vi "Get Next.vi"(0 "Conditional in":refnum<class "Case Structure.lvclass">, 1 "Linked List Ref":refnum<data-value>, 5 "Active Unique ID":string, 9 "Active Element Index":i32, 11 "error in (no error)":errorcluster) -> (3 "Linked List Ref out":refnum<data-value>, 4 "Executioner out":refnum<class "Executioner.lvclass">, 6 "Active Unique ID out":string, 8 "Test Executive Ref out":refnum<data-value>, 10 "Active Element Index out":i32, 12 "Found":bool, 13 "Complete":bool, 14 "Stop":bool, 15 "error out":errorcluster)   [LabVIEW 2017, in "Custom Type Test Executive.lvlib" / "Case Structure.lvclass"]
uses:
  <vilib>/gpm_packages/@cs/test-executive/Source/Custom Type Test Executive/Case Structure/Case Structure.lvclass
  C:/Program Files/National Instruments/LabVIEW 2017/vi.lib/gpm_packages/@cs/test-executive/Source/Test Executive/Executioner/Executioner.lvclass
  <vilib>/gpm_packages/@cs/test-executive/Source/Test Executive/Executioner/Executioner.lvclass
  <vilib>/gpm_packages/@cs/linked-list/Source/Linked List/ILinkedList/ILinked List.lvclass
  <vilib>/gpm_packages/@cs/test-executive/Source/Test Executive/ITestExecutive/ITest Executive.lvclass
  <vilib>/gpm_packages/@cs/data-type-serializer/source/Boolean/Boolean.lvclass/Boolean.ctl
  <vilib>/gpm_packages/@cs/run-time-assertions/Source/Assert/Assert.lvclass
  <vilib>/gpm_packages/@cs/data-type-serializer/source/String 1D/String 1D.lvclass/String 1D.ctl
  <vilib>/gpm_packages/@cs/data-type-serializer/source/Assertion 1D/Assertion 1D.lvclass/Assertion 1D.ctl
  <vilib>/gpm_packages/@cs/data-type-serializer/source/I32/I32.lvclass/I32.ctl
  <vilib>/gpm_packages/@cs/data-type-serializer/source/String/String.lvclass/String.ctl
  e3f8ce14-f829-49f2-b732-6c6bdfab1e2b.vi
  37905dbb-9ffa-4c29-9283-9b2d51775808.vi
  3e0f320b-1dba-4963-93ff-3147506816ec.vi
  cd02d659-4998-4fe8-9163-758659dc25cf.vi
  573c41b1-dd6f-44f0-b272-1a8672389ddc.vi
  138538c4-910c-479f-b7e4-eec8342ec67d.vi
  dfe7eb8f-9477-4e6f-83e2-2ac45f956d87.vi
  83fabfc2-d942-454a-aebd-5c424e9e8ceb.vi
  7aa6beab-24c8-424d-8c21-694c569c77be.vi
  c330ebbc-4213-473c-a39d-77c385c7404d.vi
  e43c0b16-206a-4550-822b-640e3cfc4d82.vi
  abd896ed-6152-4a89-b063-422a77b952e5.vi
  <vilib>/gpm_packages/@cs/data-type-serializer/source/Boolean/Boolean.lvclass
  C:/Program Files/National Instruments/LabVIEW 2017/vi.lib/gpm_packages/@cs/data-type-serializer/source/Data Type/Data Type.lvclass
  <vilib>/gpm_packages/@cs/data-type-serializer/source/Assertion 1D/Assertion 1D.lvclass
  <vilib>/gpm_packages/@cs/data-type-serializer/source/String 1D/String 1D.lvclass
  <vilib>/gpm_packages/@cs/data-type-serializer/source/I32/I32.lvclass
  <vilib>/gpm_packages/@cs/data-type-serializer/source/String/String.lvclass
  <vilib>/gpm_packages/@cs/linked-list/Source/Linked List/Linked List Ref/Linked List Ref.lvclass
  <vilib>/gpm_packages/@cs/test-executive/Source/Test Executive/Case Structure/Case Structure.lvclass
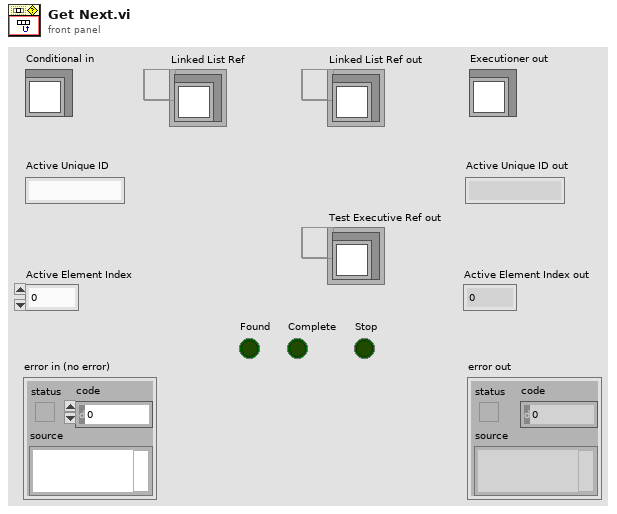
[diagram p1: front panel]
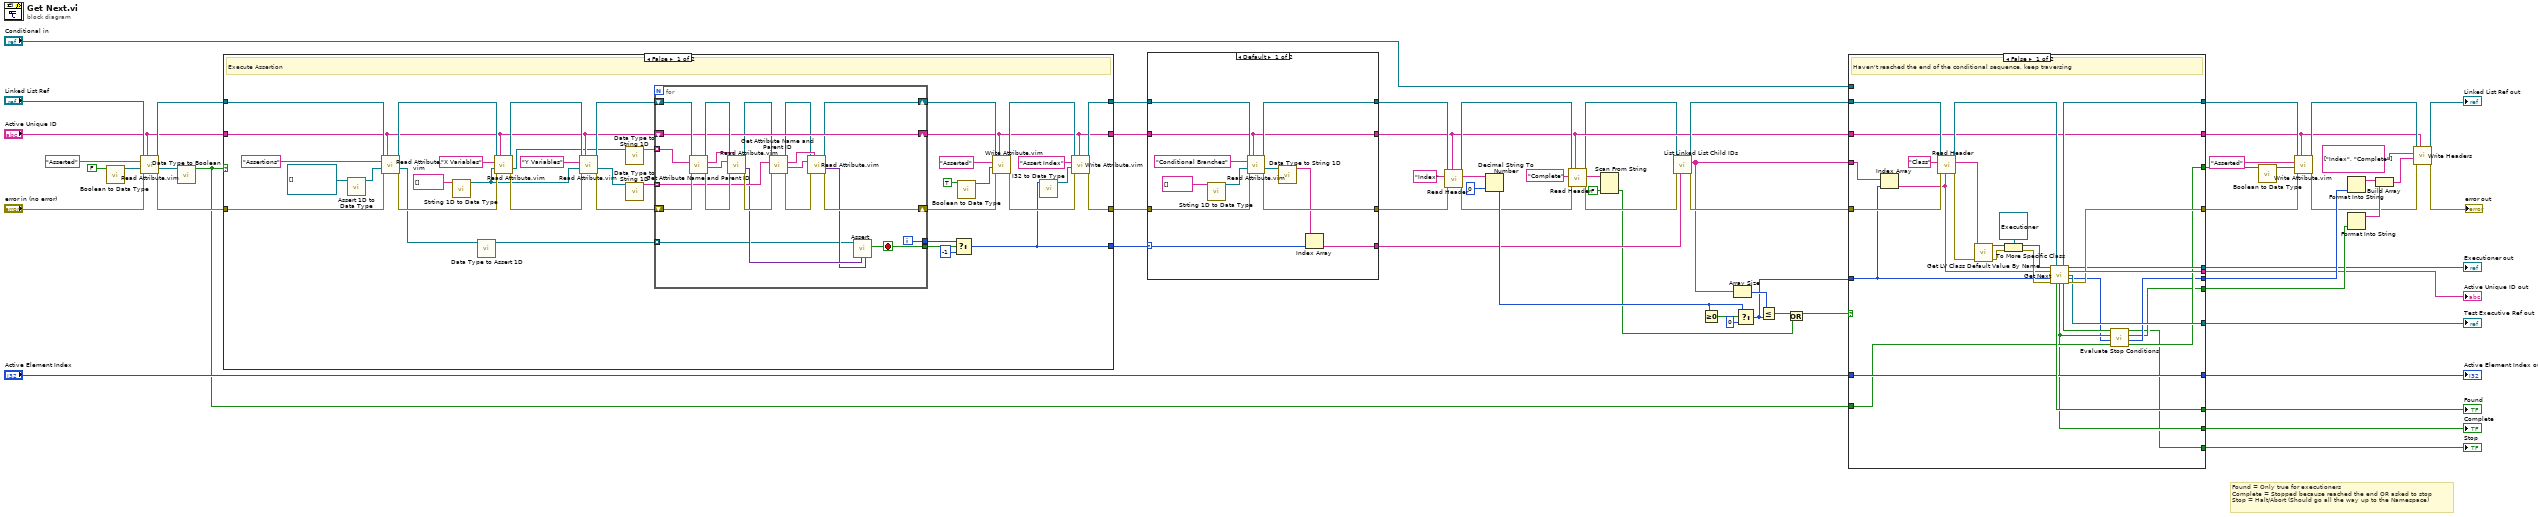
[diagram p0: block diagram]
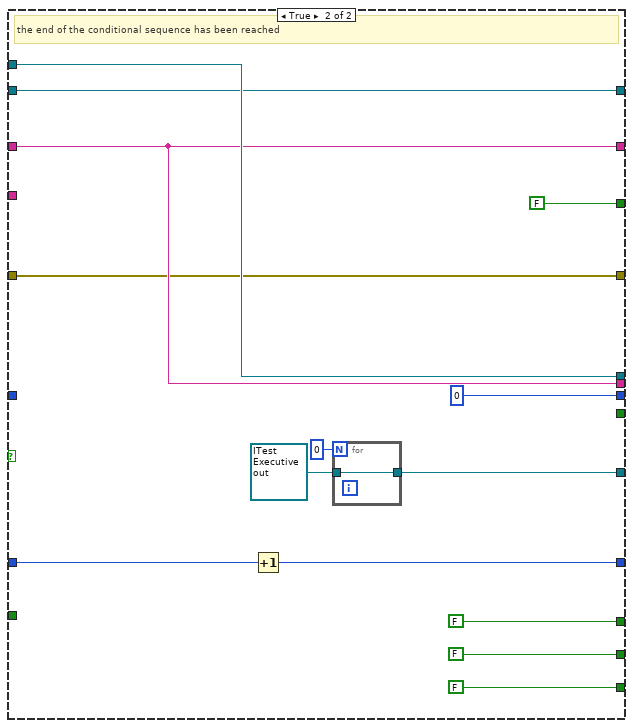
[diagram p2: hidden frame]
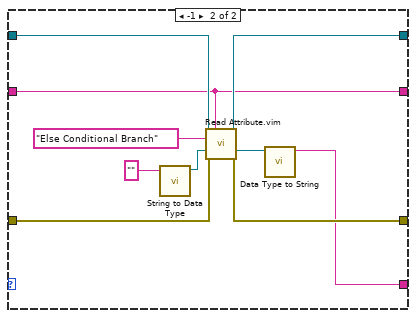
[diagram p3: hidden frame]
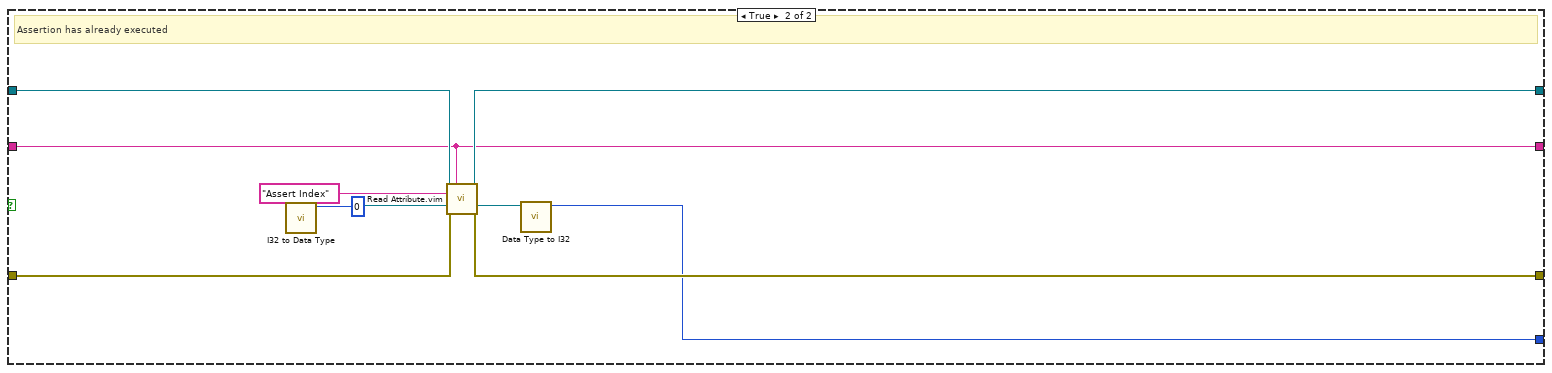
[diagram p4: hidden frame]
diagram:
  # "Found = Only true for executioners\nComplete = Stopped because reached the end OR asked to stop\nStop = Halt/Abort (Should go all the way up to the Namespace)"
  n1 = call <vilib>:"Boolean to Data Type.vi"("Boolean"=FALSE) -> ("Boolean out"=w5:refnum<class "Boolean.lvclass">)  [unwired: 9 in, 1 out]
  n2 = call "Read Attribute.vim"("Linked List Ref"="Linked List Ref", "Linked List ID"="Active Unique ID", "Attribute Name"="Asserted", "Type"=w5, "error in (no error)"="error in (no error)") -> ("Linked List Ref out"=w63:refnum<data-value>, "Attribute"=w4:refnum<class "Boolean.lvclass">, "error out"=w62:errorcluster)  [unwired: 5 in, 3 out]
  n3 = call <vilib>:"Data Type to Boolean.vi"("Data Type"=w4) -> ("Boolean out"=w3:bool)  [unwired: 9 in, 1 out]
  n4 = case shown="False" w3 {
    tunnel: "Active Unique ID" -> [w83 w129]
    tunnel: [w93 w132] -> w42
    tunnel: [w91 w130] -> w44
    tunnel: w63 -> [w97 w133]
    tunnel: w62 -> [w96 w131]
    tunnel: [w82 w129] -> w46
    tunnel: [w66 w125] -> w41
    frame False {
      # "Execute Assertion"
      n5 = call <vilib>:"Assert 1D to Data Type.vi"("Assert 1D"=refnum<class "Assert.lvclass">[] [] ("Assertions")) -> ("Boolean out"=w78:refnum<class "Assertion 1D.lvclass">)  [unwired: 9 in, 1 out]
      n6 = call "Read Attribute.vim"("Linked List Ref"=w97, "Linked List ID"=w83, "Attribute Name"="Assertions", "Type"=w78, "error in (no error)"=w96) -> ("Linked List Ref out"=w101:refnum<data-value>, "Attribute"=w76:refnum<class "Assertion 1D.lvclass">, "error out"=w100:errorcluster)  [unwired: 5 in, 3 out]
      n7 = call <vilib>:"Strting 1D to Data Type.vi"("String 1D"=string[] []) -> ("Boolean out"=w74:refnum<class "String 1D.lvclass">)  [unwired: 9 in, 1 out]
      n8 = call <vilib>:"Data Type to Assert 1D.vi"("Data Type"=w76) -> ("Assert 1D out"=w75:refnum<class "Assert.lvclass">[])  [unwired: 9 in, 1 out]
      n9 = call "Read Attribute.vim"("Linked List Ref"=w101, "Linked List ID"=w83, "Attribute Name"="X Variables", "Type"=w74, "error in (no error)"=w100) -> ("Linked List Ref out"=w88:refnum<data-value>, "Attribute"=w72:refnum<class "String 1D.lvclass">, "error out"=w89:errorcluster)  [unwired: 5 in, 3 out]
      n10 = call "Read Attribute.vim"("Linked List Ref"=w88, "Linked List ID"=w83, "Attribute Name"="Y Variables", "Type"=w74, "error in (no error)"=w89) -> ("Linked List Ref out"=w87:refnum<data-value>, "Attribute"=w70:refnum<class "String 1D.lvclass">, "error out"=w85:errorcluster)  [unwired: 5 in, 3 out]
      n11 = call <vilib>:"Data Type to String 1D.vi"("Data Type"=w72) -> ("String 1D out"=w71:string[])  [unwired: 9 in, 1 out]
      n12 = call <vilib>:"Data Type to String 1D.vi"("Data Type"=w70) -> ("String 1D out"=w69:string[])  [unwired: 9 in, 1 out]
      n13 = for {
        shift-right: [w109] -> w86
        shift-left: w87 -> [w124]
        shift-right: [w108] -> w84
        shift-left: w85 -> [w122]
        tunnel: w69 -> [w110] mode=indexing
        tunnel: w71 -> [w120] mode=indexing
        tunnel: w75 -> [w103] mode=indexing
        shift-right: [w117] -> w82
        shift-left: w83 -> [w117]
        tunnel: [w107] -> w80
        tunnel: [w106] -> w79
        i -> [w107]
        stop <- w106 stop-if-true
        n14 = call <vilib>:"Get Attribute Name and Parent ID.vi"("error in (no error)"=w122, "Tag"=w120, "Linked List Ref"=w124) -> ("error out"=w121:errorcluster, "Attribute Name"=w119:string, "Linked List ID"=w118:string, "Linked List Ref out"=w123:refnum<data-value>)  [unwired: 5 in]
        n15 = call "Read Attribute.vim"("Linked List Ref"=w123, "Linked List ID"=w118, "Attribute Name"=w119, "error in (no error)"=w121) -> ("Linked List Ref out"=w111:refnum<data-value>, "Attribute"=w105:variant, "error out"=w112:errorcluster)  [unwired: 6 in, 3 out]
        n16 = call <vilib>:"Get Attribute Name and Parent ID.vi"("error in (no error)"=w112, "Tag"=w110, "Linked List Ref"=w111) -> ("error out"=w114:errorcluster, "Attribute Name"=w115:string, "Linked List ID"=w116:string, "Linked List Ref out"=w113:refnum<data-value>)  [unwired: 5 in]
        n17 = call "Read Attribute.vim"("Linked List Ref"=w113, "Linked List ID"=w116, "Attribute Name"=w115, "error in (no error)"=w114) -> ("Linked List Ref out"=w109:refnum<data-value>, "Attribute"=w104:variant, "error out"=w108:errorcluster)  [unwired: 6 in, 3 out]
        n18 = call-dynamic "Assert.vi"("Variable Y"=w104, "Variable X"=w105, "Assert in"=w103) -> ("Assert?"=w106:bool)  [unwired: 8 in]
      }
      n19 = Select(t=w80, s=w79, f=-1) -> (s? t:f=w66:i32)
      n20 = call <vilib>:"Boolean to Data Type.vi"("Boolean"=TRUE) -> ("Boolean out"=w68:refnum<class "Boolean.lvclass">)  [unwired: 9 in, 1 out]
      n21 = call "Write Attribute.vim"("Linked List ID"=w82, "error in (no error)"=w84, "Attribute"=w68, "Attribute Name"="Asserted", "Linked List Ref"=w86) -> ("error out"=w92:errorcluster, "Linked List Ref out"=w94:refnum<data-value>)  [unwired: 3 in, 2 out]
      n22 = call <vilib>:"I32 to Data Type.vi"("I32"=w66) -> ("Boolean out"=w65:refnum<class "I32.lvclass">)  [unwired: 9 in, 1 out]
      n23 = call "Write Attribute.vim"("Linked List ID"=w82, "error in (no error)"=w92, "Attribute"=w65, "Attribute Name"="Assert Index", "Linked List Ref"=w94) -> ("error out"=w91:errorcluster, "Linked List Ref out"=w93:refnum<data-value>)  [unwired: 3 in, 2 out]
    }
    frame True {
      # "Assertion has already executed"
      n24 = call <vilib>:"I32 to Data Type.vi"("I32"=0) -> ("Boolean out"=w127:refnum<class "I32.lvclass">)  [unwired: 9 in, 1 out]
      n25 = call "Read Attribute.vim"("Linked List Ref"=w133, "Linked List ID"=w129, "Attribute Name"="Assert Index", "Type"=w127, "error in (no error)"=w131) -> ("Linked List Ref out"=w132:refnum<data-value>, "Attribute"=w126:refnum<class "I32.lvclass">, "error out"=w130:errorcluster)  [unwired: 5 in, 3 out]
      n26 = call <vilib>:"Data Type to I32.vi"("Data Type"=w126) -> ("I32 out"=w125:i32)  [unwired: 9 in, 1 out]
    }
  }
  n27 = case shown="Default" w41 {
    selector: w41 -> [w141 _]
    tunnel: w46 -> [w139 w151]
    tunnel: [w146 w156] -> w45
    tunnel: w44 -> [w145 w155]
    tunnel: [w144 w154] -> w43
    tunnel: w42 -> [w143 w153]
    tunnel: [w140 w147] -> w40
    tunnel: [w139 w151] -> w32
    frame Default {
      n28 = call <vilib>:"Strting 1D to Data Type.vi"("String 1D"=string[] []) -> ("Boolean out"=w137:refnum<class "String 1D.lvclass">)  [unwired: 9 in, 1 out]
      n29 = call "Read Attribute.vim"("Linked List Ref"=w143, "Linked List ID"=w139, "Attribute Name"="Conditional Branches", "Type"=w137, "error in (no error)"=w145) -> ("Linked List Ref out"=w144:refnum<data-value>, "Attribute"=w136:refnum<class "String 1D.lvclass">, "error out"=w146:errorcluster)  [unwired: 5 in, 3 out]
      n30 = call <vilib>:"Data Type to String 1D.vi"("Data Type"=w136) -> ("String 1D out"=w135:string[])  [unwired: 9 in, 1 out]
      n31 = Index Array(array=w135, index=w141) -> (element=w140:string)
    }
    frame -1 {
      n32 = call <vilib>:"String to Data Type.vi"("String"="") -> ("Boolean out"=w149:refnum<class "String.lvclass">)  [unwired: 9 in, 1 out]
      n33 = call "Read Attribute.vim"("Linked List Ref"=w153, "Linked List ID"=w151, "Attribute Name"="Else Conditional Branch", "Type"=w149, "error in (no error)"=w155) -> ("Linked List Ref out"=w154:refnum<data-value>, "Attribute"=w148:refnum<class "String.lvclass">, "error out"=w156:errorcluster)  [unwired: 5 in, 3 out]
      n34 = call <vilib>:"Data Type to String.vi"("Data Type"=w148) -> ("String out"=w147:string)  [unwired: 9 in, 1 out]
    }
  }
  n35 = call <vilib>:"Read Header.vi"("Linked List ID"=w32, "error in (no error)"=w45, "Header Name"="Index" ("Attribute Name"), "Linked List Ref"=w43) -> ("error out"=w30:errorcluster, "Header Value"=w51:string, "Linked List Ref out"=w33:refnum<data-value>)  [unwired: 4 in, 1 out]
  n36 = Decimal String To Number(string=w51, default (0L)=0 ("Attribute")) -> (number=w58:i32)  [unwired: 1 in, 1 out]
  n37 = call <vilib>:"Read Header.vi"("Linked List ID"=w32, "error in (no error)"=w30, "Header Name"="Complete" ("Attribute Name"), "Linked List Ref"=w33) -> ("error out"=w29:errorcluster, "Header Value"=w35:string, "Linked List Ref out"=w31:refnum<data-value>)  [unwired: 4 in, 1 out]
  n38 = Scan From String(input string=w35, default 1=FALSE) -> (output 1=w27:bool)  [unwired: 3 in, 3 out]
  n39 = call <vilib>:"List Linked List Child IDs.vi"("Linked List ID"=w40, "error in (no error)"=w29, "Linked List Ref"=w31) -> ("error out"=w56:errorcluster, "Child IDs"=w55:string[], "Linked List Ref out"=w57:refnum<data-value>)  [unwired: 6 in]
  n40 = Greater Or Equal To 0?(x=w58) -> (x >= 0?=w61:bool)
  n41 = Array Size(array=w55) -> (size(s)=w59:i32)
  n42 = Select(t=w58, s=w61, f=0) -> (s? t:f=w54:i32)
  n43 = Less Or Equal?(x=w59, y=w54) -> (x <= y?=w39:bool)
  n44 = Or(x=w39, y=w27) -> (x .or. y?=w28:bool)
  n45 = case shown="False" w28 {
    tunnel: [w176 w189] -> w24
    tunnel: w57 -> [w178 w189]
    tunnel: [w172 w188] -> w22
    tunnel: w56 -> [w180 w188]
    tunnel: w55 -> [w169 _]
    tunnel: w54 -> [w168 _]
    tunnel: [w159 0 ("Active Element Index out")] -> w53
    tunnel: [w165 w197] -> w8
    tunnel: [w175 w193] -> w7
    tunnel: [w174 FALSE ("Found")] -> w12
    tunnel: [w161 FALSE] -> w11
    tunnel: [w157 FALSE] -> w10
    tunnel: "Conditional in" -> [_ w197]
    tunnel: w32 -> [w171 w193]
    tunnel: [w171 w193] -> w21
    tunnel: "Active Element Index" -> [w170 w195]
    tunnel: [w170 w194] -> w13
    tunnel: [w166 w190] -> w14
    tunnel: [w158 _] -> w38
    tunnel: [w163 FALSE] -> w2
    tunnel: w3 -> [w162 _]
    frame False {
      # "Haven't reached the end of the conditional sequence, keep traversing"
      n46 = Index Array(array=w169, index=w168) -> (element=w167:string)
      n47 = call <vilib>:"Read Header.vi"("Linked List ID"=w167, "error in (no error)"=w180, "Header Name"="Class", "Linked List Ref"=w178) -> ("error out"=w173:errorcluster, "Header Value"=w186:string, "Linked List Ref out"=w177:refnum<data-value>)  [unwired: 4 in, 1 out]
      n48 = call <vilib>:"Get LV Class Default Value By Name.vi"("error in (no error)"=w173, "class name"=w186) -> ("error out"=w182:errorcluster, "object"=w185:refnum<class>)  [unwired: 8 in]
      n49 = To More Specific Class(target class=refnum<class "Executioner.lvclass"> refnum ("Test Executive.lvlib:Executioner.lvclass"), reference=w185, error in=w182) -> (specific class reference=w181:refnum<class "Executioner.lvclass">, error out=w183:errorcluster)
      n50 = call-dynamic "Get Next.vi"("Executioner in"=w181, "Linked List Ref"=w177, "Active Unique ID"=w167, "Active Element Index"=w168, "error in (no error)"=w183) -> ("Linked List Ref out"=w176:refnum<data-value>, "Executioner out"=w165:refnum<class "Executioner.lvclass">, "Active Unique ID out"=w175:string, "Test Executive Ref out"=w166:refnum<data-value>, "Active Element Index out"=w160:i32, "Found"=w174:bool, "Complete"=w161:bool, "Stop"=w164:bool, "error out"=w172:errorcluster)  [unwired: 2 in]
      n51 = call <vilib>:"Evaluate Stop Conditions.vi"("Assert"=w162, "Index"=w160, "Complete"=w161, "Stop"=w164) -> ("Asserted"=w163:bool, "Index out"=w159:i32, "Completed"=w158:bool, "Stop out"=w157:bool)  [unwired: 4 in]
    }
    frame True {
      # "the end of the conditional sequence has been reached"
      n52 = Increment(x=w195) -> (x+1=w194:i32)
      n53 = for {
        N: 0 -> [_]
        tunnel: refnum<data-value> refnum ("Test Executive Ref out") -> [w201]
        tunnel: [w201] -> w190
      }
    }
  }
  "Executioner out" <- w8
  "Active Unique ID out" <- w7
  "Active Element Index out" <- w13
  "Found" <- w12
  "Complete" <- w11
  "Stop" <- w10
  "Test Executive Ref out" <- w14
  n54 = call <vilib>:"Boolean to Data Type.vi"("Boolean"=w2) -> ("Boolean out"=w1:refnum<class "Boolean.lvclass">)  [unwired: 9 in, 1 out]
  n55 = call "Write Attribute.vim"("Linked List ID"=w21, "error in (no error)"=w22, "Attribute"=w1, "Attribute Name"="Asserted", "Linked List Ref"=w24) -> ("error out"=w23:errorcluster, "Linked List Ref out"=w25:refnum<data-value>)  [unwired: 3 in, 2 out]
  n56 = Format Into String(w53) -> (resulting string=w48:string)  [unwired: 3 in, 1 out]
  n57 = Format Into String(w38) -> (resulting string=w37:string)  [unwired: 3 in, 1 out]
  n58 = Build Array(w48, w37) -> (w47:string[])
  n59 = call <vilib>:"Write Headers.vi"("Linked List ID"=w21, "error in (no error)"=w23, "Header Values"=w47, "Header Names"=string[] ["Index", "Complete"], "Linked List Ref"=w25) -> ("error out"=→"error out":errorcluster, "Linked List Ref out"=→"Linked List Ref out":refnum<data-value>)  [unwired: 5 in]
